vi "2D to XY.vi"(8 "error in (no error)":errorcluster, 10 "X Array":dbl[](array[numeric]), 11 "2D Z Array":dbl[][](array[numeric])) -> (0 "error out":errorcluster, 3 "XY-data out":cluster{"X-array":dbl[], "Y-array":dbl[]}[](array[cluster]) {"Y-array" format="%.2p"; "X-array" format="%.2p"})   [LabVIEW 2019, in "xy_utilities.lvlib"]
doc: "Convert <b>2D Z Array</b> and <b>X Array</b> to Array of <b>XY-Data</b> (where <b>XY = XZ</b>)"
uses:
  xy_utilities.lvlib
panel:
  out "Numeric":i32
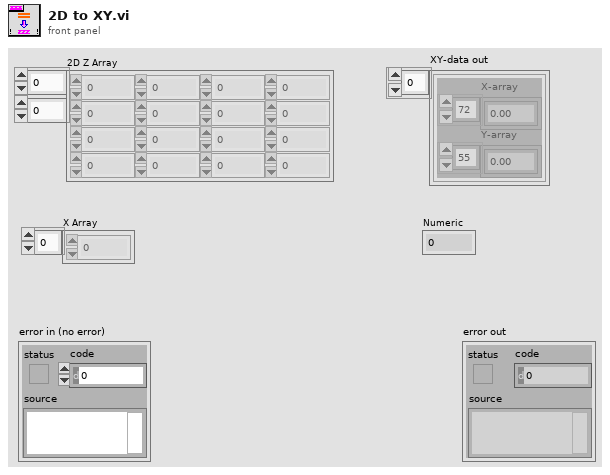
[diagram p1: front panel]
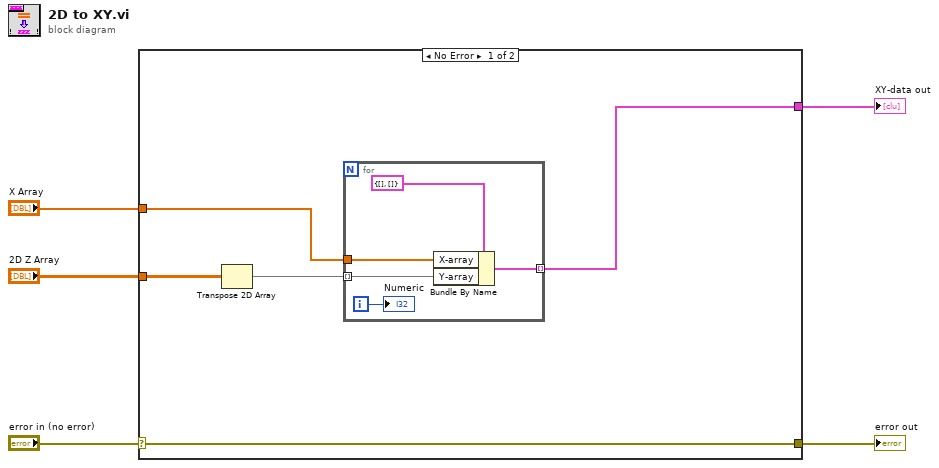
[diagram p0: block diagram]
diagram:
  n1 = case shown="No Error" "error in (no error)" {
    selector: "error in (no error)" -> [w10 w16]
    tunnel: [w10 w16] -> w4
    tunnel: [w8 _] -> w3
    tunnel: "2D Z Array" -> [w7 _]
    tunnel: "X Array" -> [w9 _]
    frame No Error {
      n2 = Transpose 2D Array(2D array=w7) -> (transposed array=w6:dbl[][])
      n3 = for {
        tunnel: w6 -> [w14] mode=indexing
        tunnel: w9 -> [w12]
        tunnel: [w13] -> w8 mode=indexing
        i -> [w11]
        n4 = Bundle By Name(cluster=cluster{"X-array":dbl[], "Y-array":dbl[]} {"X-array"=[], "Y-array"=[]}, "X-array"=w12, "Y-array"=w14) -> (w13:cluster{"X-array":dbl[], "Y-array":dbl[]})
        "Numeric" <- w11
      }
    }
    frame Error {
    }
  }
  "error out" <- w4
  "XY-data out" <- w3
